vi "Dereferncing 2D Array Pointer.vi"(8 "error in (no error)":errorcluster, 9 "2D Array Pointer":u64, 10 "numberOfSamples":u32, 11 "numberOfEncoder":u32) -> (0 "error out":errorcluster, 3 "Array Data":u16[][](array[numeric]))   [LabVIEW 2017]
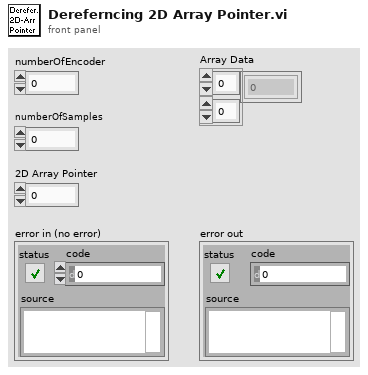
[diagram p1: front panel]
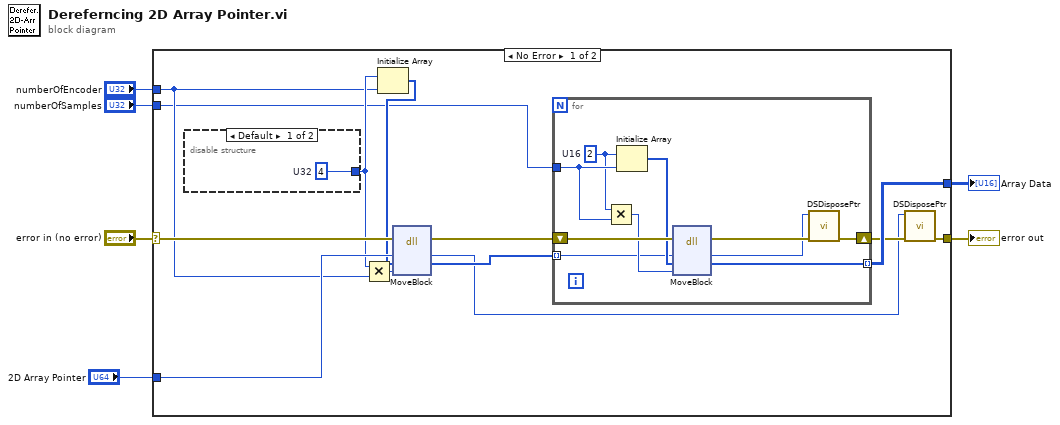
[diagram p0: block diagram]
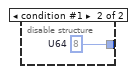
[diagram p2: hidden frame]
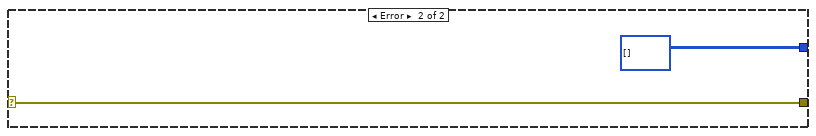
[diagram p3: hidden frame]
diagram:
  n1 = case shown="No Error" "error in (no error)" {
    selector: "error in (no error)" -> [w17 w32]
    tunnel: "numberOfSamples" -> [w9 _]
    tunnel: "numberOfEncoder" -> [w13 _]
    tunnel: "2D Array Pointer" -> [w15 _]
    tunnel: [w19 w32] -> w3
    tunnel: [w18 u16[][] []] -> w2
    frame No Error {
      n2 = disable-structure shown="Default" {
        disable-tunnel: [w20 w21] -> w14
        frame condition #0 (active) {
          w20 = u32 4  # U32
        }
        frame condition #1 {
          w21 = u64 8  # U64
        }
      }
      n3 = Multiply(x=w14, y=w13) -> (x*y=w12:u32)
      n4 = Initialize Array(w14, w13) -> (w11:u32[])
      n5 = dll-call lib="LabVIEW" fn="MoveBlock"(error in=w17, "source"=w15, "dest"=w11, "size"=w12) -> (error out=w16:errorcluster, "source"=w7:i64, "dest"=w10:u32[])  [unwired: 4 in, 1 out]
      n6 = for {
        tunnel: [w30] -> w18 mode=indexing
        shift-right: [w24] -> w8
        shift-left: w16 -> [w31]
        tunnel: w10 -> [w23] mode=indexing
        tunnel: w9 -> [w29]
        w28 = u16 2  # U16
        n7 = Multiply(x=w28, y=w29) -> (x*y=w27:u32)
        n8 = Initialize Array(w28, w29) -> (w26:u16[])
        n9 = dll-call lib="LabVIEW" fn="MoveBlock"(error in=w31, "source"=w23, "dest"=w26, "size"=w27) -> (error out=w25:errorcluster, "source"=w22:i64, "dest"=w30:u16[])  [unwired: 4 in, 1 out]
        n10 = call <vilib>:"DSDisposePtr.vi"("error in (no error)"=w25, "Pointer"=w22) -> ("error out"=w24:errorcluster)  [unwired: 9 in]
      }
      n11 = call <vilib>:"DSDisposePtr.vi"("error in (no error)"=w8, "Pointer"=w7) -> ("error out"=w19:errorcluster)  [unwired: 9 in]
    }
    frame Error {
    }
  }
  "error out" <- w3
  "Array Data" <- w2
